vi "Semaphore Timed Wait (absolute timespec).vi"(8 "error in (no error)":errorcluster, 10 "absolute timeout (timespec)":cluster{"sec":u64, "nsec":u64}, 11 "Semaphore in":T1) -> (0 "error out":errorcluster, 2 "timed out?":bool, 3 "Semaphore out":T1)   [LabVIEW 2016, in "Linux RT IPC.POSIX Threads.lvlib" / "Semaphore.lvclass"]
doc: "Calls sem_timedwait() on the semaphore object encapsulated by Semaphore.\n\nThis VI attempts to decrement the value of the semaphore by 1 within a timeout period. If the semaphore can be decremented within the timeout period, this VI returns indicating it was successful. Otherwise, this VI returns indicating the semaphore was never set.\n\nTo provide a valid absolute timeout, query the Realtime clock for the current time and offset the time by the desired timeout duration.\n\nRefer to online POSIX documentation for more information."
uses:
  Semaphore.lvclass
  Controls/reference.ctl
  C:/Git/SourceTree/LinuxRT-IPC/Source/POSIX Threads/Classes/POSIX Thread Object/POSIX Thread Object.lvclass
  POSIX Thread Object/POSIX Thread Object.lvclass/POSIX Thread Object.ctl
  POSIX Thread Object/Private VIs/libpthread path.vi
  <vilib>/NI/NI Linux RT Utilities/VIs/Public/Convert Types/convert timespec 64 to timespec 32.vi
  POSIX Thread Object/Private VIs/get pthread error.vi
  <vilib>/NI/NI Linux RT Errno/VIs/Public/SubVIs/errno enum to number.vi
  <vilib>/NI/NI Linux RT Errno/VIs/Public/Get Errno Value for Calling Thread.vi
  POSIX Thread Object/POSIX Thread Object.lvclass
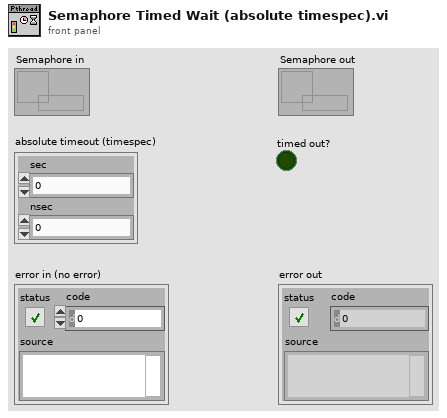
[diagram p1: front panel]
types:
  T1 = typedef "Linux RT IPC.POSIX Threads.lvlib/Semaphore.lvclass/reference.ctl" = refnum<data-value>
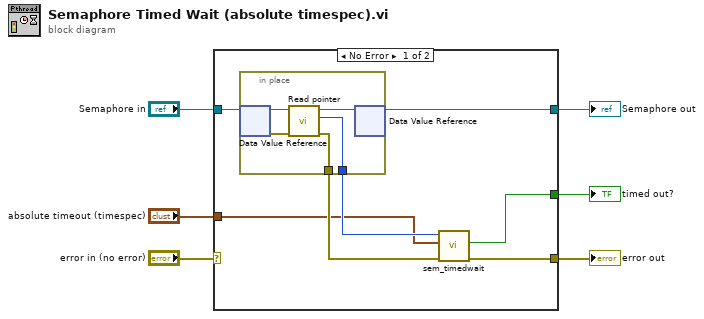
[diagram p0: block diagram]
diagram:
  n1 = case shown="No Error" "error in (no error)" {
    selector: "error in (no error)" -> [_ w19]
    tunnel: "Semaphore in" -> [w13 w20]
    tunnel: [w12 w20] -> w3
    tunnel: [w10 w19] -> w4
    tunnel: [w8 _] -> w2
    tunnel: "absolute timeout (timespec)" -> [w7 _]
    frame No Error {
      n2 = in-place {
        in-place-border: [w15] -> w11
        in-place-border: [w14] -> w9
        n3 = in-place-dvr #1(w13) -> (w18:refnum<class "Semaphore.lvclass">, w17:errorcluster)
        n4 = call "Read pointer.vi"("error in (no error)"=w17, "POSIX Thread Object in"=w18) -> ("error out"=w15:errorcluster, "pointer"=w14:u64, "POSIX Thread Object out"=w16:refnum<class "Semaphore.lvclass">)  [unwired: 7 in]
        n5 = in-place-dvr #1(w16) -> (w12:T1)  [unwired: 1 out]
      }
      n6 = call "sem_timedwait.vi"("error in (no error)"=w11, "absolute timeout"=w7, "sempahore ptr in"=w9) -> ("error out"=w10:errorcluster, "timed out?"=w8:bool)  [unwired: 6 in, 1 out]
    }
    frame Error {
    }
  }
  "error out" <- w4
  "Semaphore out" <- w3
  "timed out?" <- w2
